vi "Start Sync.vi"(8 "error in (no error)":errorcluster, 11 "gRPC Server in":refnum<class "MeasurementPluginService.lvclass">) -> (0 "error out":errorcluster, 3 "gRPC Server out":refnum<class "MeasurementPluginService.lvclass">)   [LabVIEW 2020, in "MeasurementLink Measurement Server.lvlib" / "MeasurementPluginService.lvclass"]
uses:
  MeasurementPluginService.lvclass
  C:/dev/measurementlink-labview/Source/Runtime/MeasurementLink Measurement Server Internal/RPC Service/MeasurementService/MeasurementService.lvclass
  MeasurementLink Measurement Server Internal/RPC Service/MeasurementService/MeasurementService.lvclass/MeasurementService.ctl
  MeasurementLink Measurement Server Internal/RPC Messages/ni_measurementlink_measurement_v1_GetMetadataResponse.ctl
  MeasurementLink Measurement Server Internal/RPC Messages/ni_measurementlink_measurement_v1_MeasurementDetails.ctl
  MeasurementLink Measurement Server Internal/RPC Messages/ni_measurementlink_measurement_v1_MeasurementSignature.ctl
  MeasurementLink Measurement Server Internal/RPC Messages/ni_measurementlink_measurement_v1_ConfigurationParameter.ctl
  MeasurementLink Measurement Server Internal/RPC Messages/ni_measurementlink_measurement_v1_ConfigurationParameter_AnnotationsEntry.ctl
  MeasurementLink Measurement Server Internal/RPC Messages/google_protobuf_Any.ctl
  MeasurementLink Measurement Server Internal/RPC Messages/ni_measurementlink_measurement_v1_Output.ctl
  MeasurementLink Measurement Server Internal/RPC Messages/ni_measurementlink_measurement_v1_UserInterfaceDetails.ctl
  <vilib>/gRPC/LabVIEW gRPC Library/Server API/typeDefs/gRPC Status Code.ctl
  MeasurementPluginService.lvclass/MeasurementPluginService.ctl
  MeasurementLink Measurement Server Internal/RPC Service/MeasurementService/MeasurementService.lvclass
  MeasurementLink Measurement Server Internal/MeasurementLink Measurement Server Internal.lvlib
  MeasurementLink Measurement Server.lvlib
  <vilib>/gRPC/LabVIEW gRPC Library/grpc-lvsupport-release.lvlib
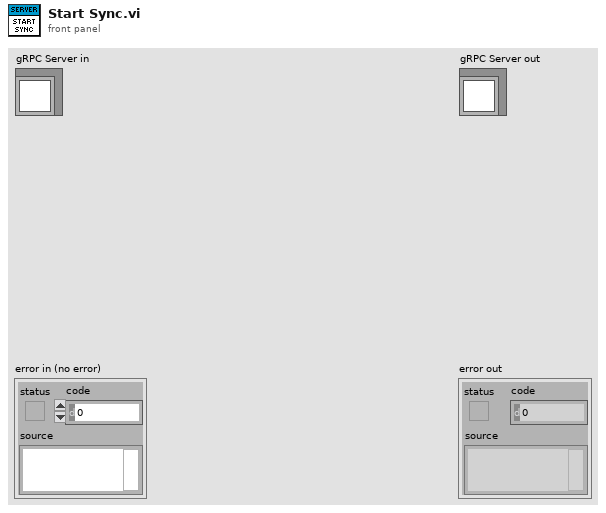
[diagram p1: front panel]
types:
  T1 = typedef "MeasurementLink Measurement Server Internal.lvlib/ni_measurementlink_measurement_v1_MeasurementSignature.ctl" = cluster{"configuration_parameters_message_type":string, "configuration_parameters":T2[], "configuration_defaults":T4, "outputs_message_type":string, "outputs":T5[]}
  T2 = typedef "MeasurementLink Measurement Server Internal.lvlib/ni_measurementlink_measurement_v1_ConfigurationParameter.ctl" = cluster{"field_number":i32, "type":i32, "name":string, "repeated":bool, "annotations":T3[]}
  T3 = typedef "MeasurementLink Measurement Server Internal.lvlib/ni_measurementlink_measurement_v1_ConfigurationParameter_AnnotationsEntry.ctl" = cluster{"key":string, "value":string}
  T4 = typedef "MeasurementLink Measurement Server Internal.lvlib/google_protobuf_Any.ctl" = cluster{"type_url":string, "value":u8[]}
  T5 = typedef "MeasurementLink Measurement Server Internal.lvlib/ni_measurementlink_measurement_v1_Output.ctl" = cluster{"field_number":i32, "type":i32, "name":string, "repeated":bool}
  T6 = typedef "MeasurementLink Measurement Server Internal.lvlib/ni_measurementlink_measurement_v1_GetMetadataResponse.ctl" = cluster{"measurement_details":T7, "measurement_signature":T1, "user_interface_details":T8[]}
  T7 = typedef "MeasurementLink Measurement Server Internal.lvlib/ni_measurementlink_measurement_v1_MeasurementDetails.ctl" = cluster{"display_name":string, "version":string}
  T8 = typedef "MeasurementLink Measurement Server Internal.lvlib/ni_measurementlink_measurement_v1_UserInterfaceDetails.ctl" = cluster{"file_url":string}
  T9 = typedef "grpc-lvsupport-release.lvlib/gRPC Status Code.ctl" = enum16{"OK", "CANCELLED", "UNKNOWN", "INVALID_ARGUMENT", "DEADLINE_EXCEEDED", "NOT_FOUND", "ALREADY_EXISTS", "PERMISSION_DENIED", "RESOURCE_EXHAUSTED", "FAILED_PRECONDITION", "ABORTED", "OUT_OF_RANGE", "UNIMPLEMENTED", "INTERNAL", "UNAVAILABLE", "DATA_LOSS", "UNAUTHENTICATED"}
  T10 = typedef "MeasurementLink Measurement Server Internal.lvlib/MeasurementService.lvclass/Server Internal UEs.ctl" = cluster{"MeasurementService GetMetadata Internal UE":refnum<user-event>, "MeasurementService Measure Internal UE":refnum<user-event>}
  T11 = typedef "MeasurementLink Measurement Server Internal.lvlib/MeasurementService.lvclass/Server gRPC UEs.ctl" = cluster{"MeasurementService GetMetadata gRPC UE":refnum<user-event>, "MeasurementService Measure gRPC UE":refnum<user-event>}
  T12 = typedef "grpc-lvsupport-release.lvlib/grpcId.ctl" = u64
  T13 = typedef "MeasurementLink Measurement Server.lvlib/MeasurementPluginService.lvclass/Plugin Paths.ctl" = cluster{"Get Measurement Details VI Path":path, "Get Type Specializations VI Path":path, "Get UI Details VI Path":path, "Measurement Logic VI Path":path, "Measurement Configuration CTL Path":path, "Measurement Results CTL Path":path}
  T14 = typedef "grpc-lvsupport-release.lvlib/Any.ctl" = cluster{"Type Url":string, "Bytes":u8[]}
  T15 = typedef "MeasurementLink Measurement Server Internal.lvlib/ni_measurementlink_measurement_v1_MeasureResponse.ctl" = cluster{"outputs":T4}
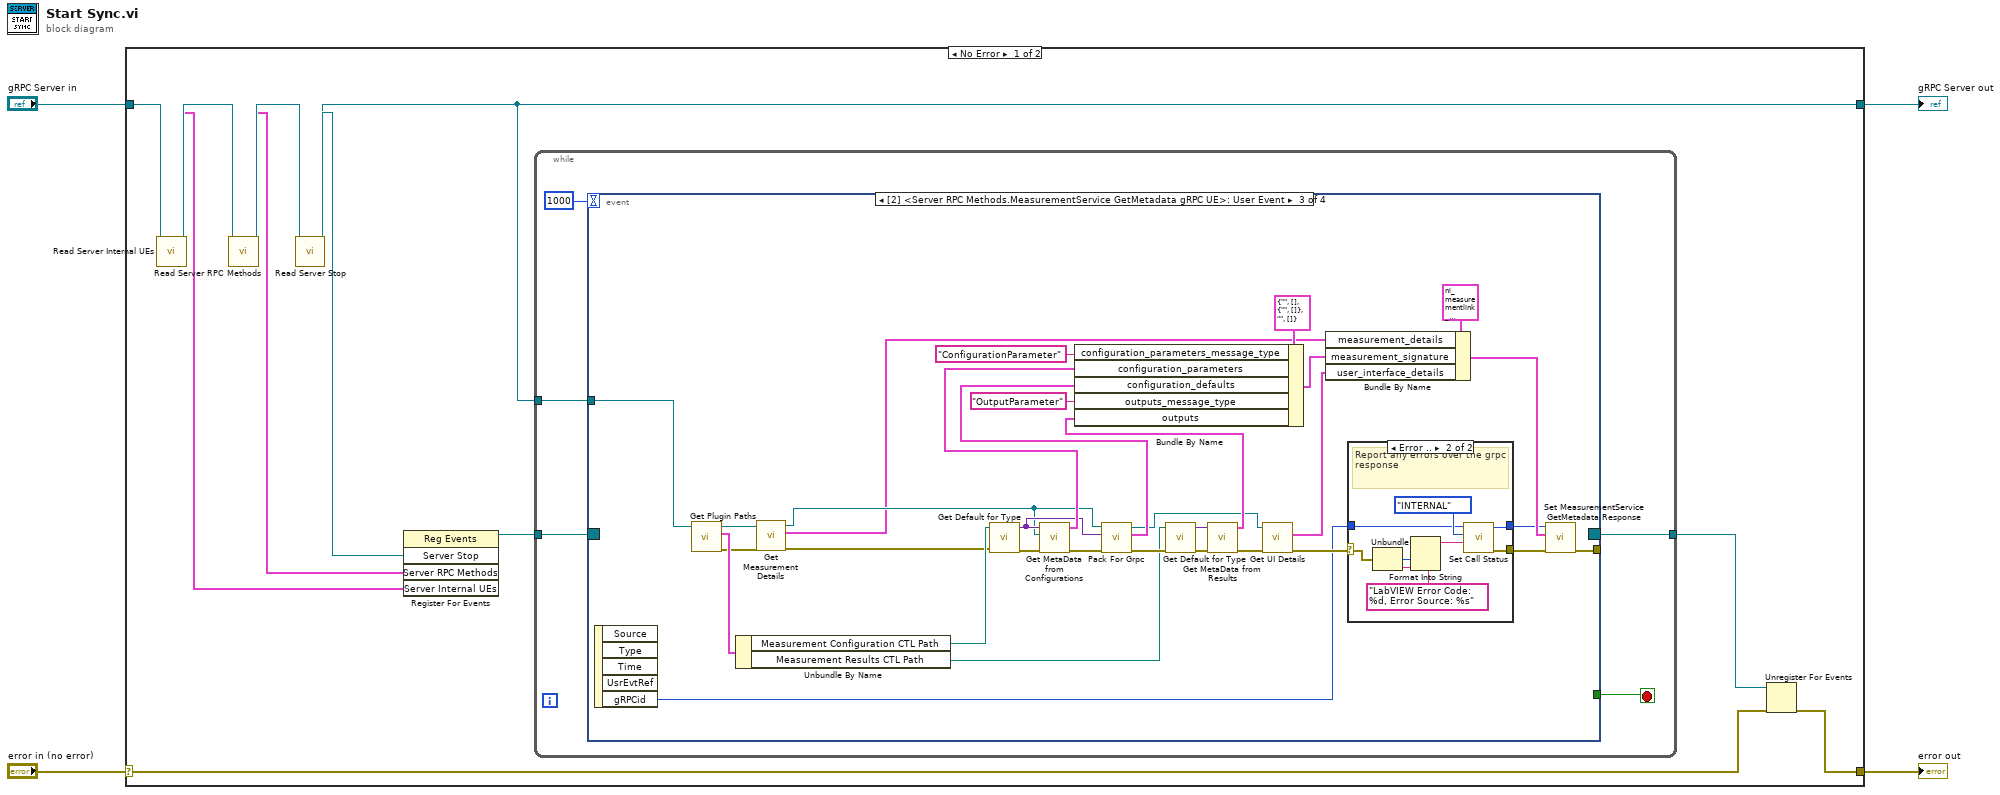
[diagram p0: block diagram]
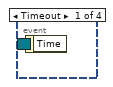
[diagram p2: hidden frame]
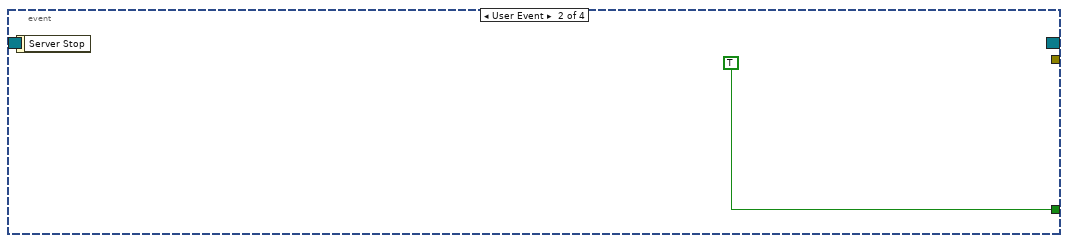
[diagram p3: hidden frame]
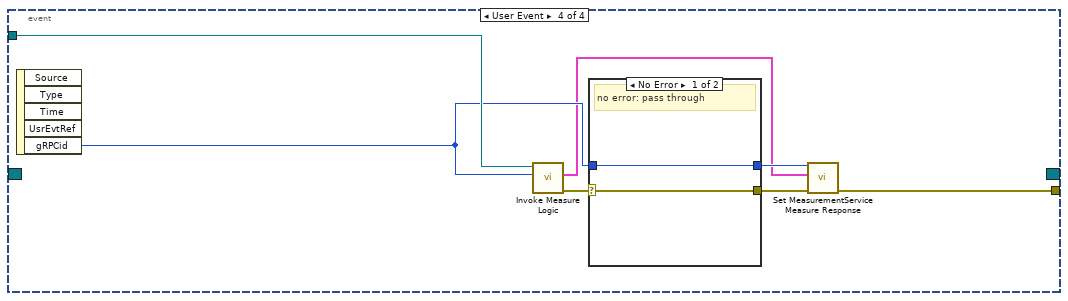
[diagram p5: hidden frame]
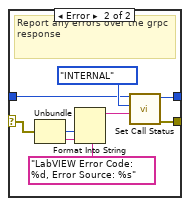
[diagram p6: hidden frame]
diagram:
  n1 = case shown="No Error" "error in (no error)" {
    selector: "error in (no error)" -> [w9 w84]
    tunnel: [w8 w84] -> w3
    tunnel: [w5 w83] -> w1
    tunnel: "gRPC Server in" -> [w15 w83]
    frame No Error {
      n2 = call "Read Server Internal UEs.vi"("SignalGeneratorService in"=w15) -> ("Server Internal UEs"=w13:T10, "SignalGeneratorService out"=w14:refnum<class "MeasurementPluginService.lvclass">)  [unwired: 8 in, 1 out]
      n3 = call "Read Server RPC Methods.vi"("SignalGeneratorService in"=w14) -> ("Server RPC Methods"=w7:T11, "SignalGeneratorService out"=w12:refnum<class "MeasurementPluginService.lvclass">)  [unwired: 8 in, 1 out]
      n4 = call-dynamic "Read Server Stop.vi"("iService in"=w12) -> ("Server Stop"=w6:refnum<user-event>, "iService out"=w5:refnum<class "MeasurementPluginService.lvclass">)  [unwired: 8 in, 1 out]
      n5 = register-events(w6, w7, w13) -> (reference out=w11:refnum<event-registration>)  [unwired: 2 in, 1 out]
      n6 = while {
        tunnel: w11 -> [w20]
        tunnel: [w18] -> w10
        tunnel: w5 -> [w16]
        stop <- w19 stop-if-true
        n7 = event "RPC Methods Event Structure" shown="[2] <Server RPC Methods.MeasurementService GetMetadata gRPC UE>: User Event" {
          selector: w20 -> [_ _ _ _]
          dyn-events: [_ _ _ _] -> w18
          timeout: 1000 -> [_ _ _ _]
          tunnel: [_ TRUE _ _] -> w19
          tunnel: w16 -> [_ _ w37 w71]
          tunnel: [_ _ w27 w65] -> _
          event Timeout {
            n8 = event-data() -> ()  [unwired: 1 in, 1 out]
          }
          event User Event {
            n9 = event-data() -> ()  [unwired: 1 in, 1 out]
          }
          event User Event {
            n10 = event-data() -> ("gRPCid"=w29:T12)  [unwired: 1 in, 4 out]
            n11 = call-dynamic "Get Plugin Paths.vi"("MeasurementService in"=w37) -> ("error out"=w24:errorcluster, "Plugin Paths"=w35:T13, "MeasurementService out"=w26:refnum<class "MeasurementPluginService.lvclass">)  [unwired: 8 in]
            n12 = Unbundle By Name(w35) -> ("Measurement Configuration CTL Path"=w34:path, "Measurement Results CTL Path"=w33:path)
            n13 = call-dynamic "Get Measurement Details.vi"("error in"=w24, "gRPC Server in"=w26) -> ("error out"=w23:errorcluster, "Measurement Details"=w22:cluster{"display_name":string, "version":string}, "gRPC Server out"=w25:refnum<class "MeasurementPluginService.lvclass">)  [unwired: 6 in, 1 out]
            n14 = call "Get Default for Type.vi"("error in (no error)"=w23, "Path of Type"=w34) -> ("error out"=w48:errorcluster, "Default for Type"=w41:variant)  [unwired: 8 in]
            n15 = call "Get MetaData from Configurations.vi"("error in"=w48, "Measurement"=w25, "Configuration Cluster"=w41) -> ("error out"=w42:errorcluster, "configuration_parameters"=w53:T2[])  [unwired: 7 in]
            n16 = call-dynamic "Pack For Grpc.vi"("error in (no error)"=w42, "Data Value"=w41, "gRPC Server in"=w25) -> ("error out"=w39:errorcluster, "Any"=w40:T14, "gRPC Server out"=w36:refnum<class "MeasurementPluginService.lvclass">)  [unwired: 6 in]
            n17 = call "Get Default for Type.vi"("error in (no error)"=w39, "Path of Type"=w33) -> ("error out"=w43:errorcluster, "Default for Type"=w44:variant)  [unwired: 8 in]
            n18 = call "Get MetaData from Results.vi"("error in"=w43, "Configuration Cluster"=w44) -> ("error out"=w49:errorcluster, "outputs"=w52:T5[])  [unwired: 8 in]
            n19 = Bundle By Name(cluster=T1 {"configuration_parameters_message_type"="", "configuration_parameters"=[], "configuration_defaults"={"type_url"="", "value"=[]}, "outputs_message_type"="", "outputs"=[]} ("ni_measurements_v1_MeasurementSignature"), "configuration_parameters_message_type"="ConfigurationParameter" ("configuration_parameters_messagetype"), "configuration_parameters"=w53, "configuration_defaults"=w40, "outputs_message_type"="OutputParameter" ("configuration_parameters_messagetype"), "outputs"=w52) -> (w46:T1)
            n20 = call-dynamic "Get UI Details.vi"("error in"=w49, "gRPC Server in"=w36) -> ("error out"=w31:errorcluster, "user_interface_details"=w38:T8[])  [unwired: 6 in, 2 out]
            n21 = Bundle By Name(cluster=T6 {"measurement_details"={"display_name"="", "version"=""}, "measurement_signature"={"configuration_parameters_message_type"="", "configuration_parameters"=[], "configuration_defaults"={"type_url"="", "value"=[]}, "outputs_message_type"="", "outputs"=[]}, "user_interface_details"=[]} ("package_templatemessage"), "measurement_details"=w22, "measurement_signature"=w46, "user_interface_details"=w38) -> (w32:T6)
            n22 = case shown="Error .." w31 {
              selector: w31 -> [w54 w58]
              tunnel: [w54 w59] -> w30
              tunnel: w29 -> [w55 w57]
              tunnel: [w55 w56] -> w28
              frame No Error {
                # "no error: pass through"
              }
              frame Error {
                # "Report any errors over the grpc response"
                n23 = Unbundle(w58) -> ("code"=w62:i32, "source"=w63:string)  [unwired: 1 out]
                n24 = Format Into String(format string="LabVIEW Error Code: %d, Error Source: %s", w62, w63) -> (resulting string=w64:string)  [unwired: 2 in, 1 out]
                n25 = call <vilib>:"Set Call Status.vi"("Details"=w64, "Status Code"=gRPC_Status_Code."INTERNAL", "gRPCid in"=w57) -> ("error out"=w59:errorcluster, "gRPCid out"=w56:T12)  [unwired: 7 in]
              }
            }
            n26 = call "Set MeasurementService GetMetadata Response.vi"("error in (no error)"=w30, "Message Data"=w32, "gRPCid in"=w28) -> ("error out"=w27:errorcluster)  [unwired: 8 in]
          }
          event User Event {
            n27 = event-data() -> ("gRPCid"=w69:T12)  [unwired: 1 in, 4 out]
            n28 = call "Invoke Measure Logic.vi"("gRPCid in"=w69, "gRPC Server in"=w71) -> ("error out"=w70:errorcluster, "Measure Response"=w66:T15)  [unwired: 8 in]
            n29 = case shown="No Error" w70 {
              selector: w70 -> [w72 w76]
              tunnel: [w72 w77] -> w68
              tunnel: w69 -> [w73 w75]
              tunnel: [w73 w74] -> w67
              frame No Error {
                # "no error: pass through"
              }
              frame Error {
                # "Report any errors over the grpc response"
                n30 = Unbundle(w76) -> ("code"=w80:i32, "source"=w81:string)  [unwired: 1 out]
                n31 = Format Into String(format string="LabVIEW Error Code: %d, Error Source: %s", w80, w81) -> (resulting string=w82:string)  [unwired: 2 in, 1 out]
                n32 = call <vilib>:"Set Call Status.vi"("Details"=w82, "Status Code"=gRPC_Status_Code."INTERNAL", "gRPCid in"=w75) -> ("error out"=w77:errorcluster, "gRPCid out"=w74:T12)  [unwired: 7 in]
              }
            }
            n33 = call "Set MeasurementService Measure Response.vi"("error in (no error)"=w68, "Message Data"=w66, "gRPCid in"=w67) -> ("error out"=w65:errorcluster)  [unwired: 8 in]
          }
        }
      }
      n34 = Unregister For Events(event registration refnum=w10, error in=w9) -> (error out=w8:errorcluster)
    }
    frame Error {
    }
  }
  "error out" <- w3
  "gRPC Server out" <- w1
